vi "Barometer Bricklet Test.vi"() -> ()   [LabVIEW 2011]
uses:
  Classes/Device/Type Definitions/Callback Option.ctl
  Classes/IP Connection/IP Connection.lvclass
  Classes/Device/Device.lvclass
  Classes/Barometer Bricklet/Barometer Bricklet.lvclass
panel:
  out "appended array":bool[](array[boolean])
  out "x-y":u32
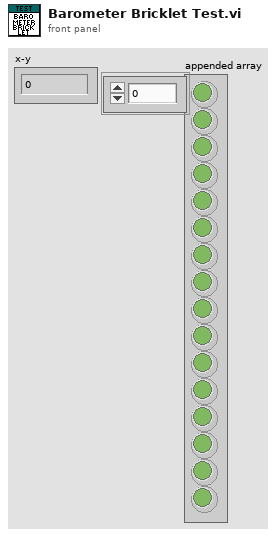
[diagram p1: front panel]
types:
  T1 = typedef "Tinkerforge.lvlib/Device.lvclass/Callback Option.ctl" = enum8{"CB off", "outside range", "inside range", "smaller", "greater"}
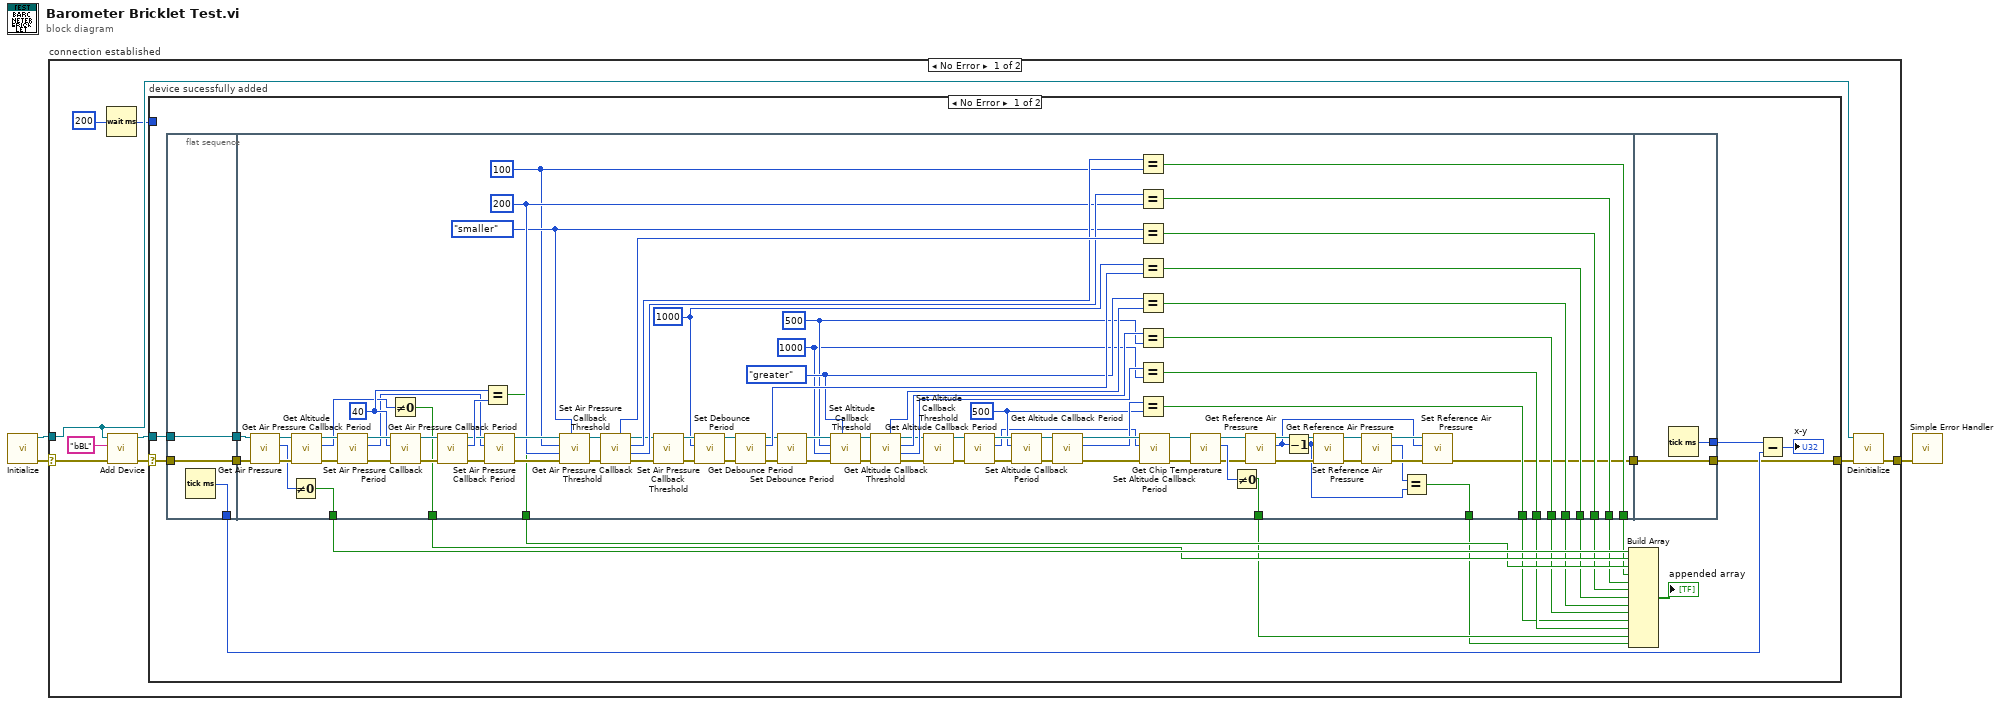
[diagram p0: block diagram]
diagram:
  n1 = call "Initialize.vi"() -> ("error out"=w1:errorcluster, "IP Connection out"=w3:refnum<class "IP Connection.lvclass">)  [unwired: 10 in]
  n2 = case "connection established" shown="No Error" w1 {
    selector: w1 -> [w8 w130]
    tunnel: w3 -> [w12 _]
    tunnel: [w4 w130] -> w2
    frame No Error {
      n3 = Wait (ms)(milliseconds to wait=u32 200) -> (millisecond timer value=w5:u32)
      n4 = call "Add Device.vi"("Error In"=w8, "Device UID"="bBL", "IP Connection"=w12) -> ("Error Out"=w7:errorcluster, "Barometer Bricklet"=w9:refnum<class "Barometer Bricklet.lvclass">)  [unwired: 7 in]
      n5 = case "device sucessfully added" shown="No Error" w7 {
        selector: w7 -> [w35 w129]
        tunnel: [w15 w129] -> w10
        tunnel: w9 -> [w34 _]
        tunnel: w5 -> [_ _]
        frame No Error {
          n6 = flat-sequence {
            tunnel: w34 -> [w37]
            tunnel: w35 -> [w38]
            tunnel: [w38] -> w32
            tunnel: [w37] -> w31
            tunnel: [w36] -> w29
            tunnel: [w43] -> w33
            tunnel: w32 -> [w126]
            tunnel: w31 -> [w125]
            tunnel: [w66] -> w27
            tunnel: [w65] -> w26
            tunnel: [w64] -> w25
            tunnel: [w63] -> w24
            tunnel: [w62] -> w23
            tunnel: [w61] -> w22
            tunnel: [w60] -> w21
            tunnel: [w59] -> w20
            tunnel: [w58] -> w19
            tunnel: [w57] -> w18
            tunnel: [w56] -> w17
            tunnel: [w42] -> w14
            tunnel: [w41] -> w13
            tunnel: [w128] -> w15
            tunnel: w33 -> [w128]
            tunnel: [w127] -> w30
            frame #0 {
              n7 = Tick Count (ms)() -> (millisecond timer value=w36:u32)
            }
            frame #1 {
              w68 = u32 500 ("period (0: off)")
              w80 = i16 1000 ("max")
              w82 = i16 500 ("min")
              w85 = Callback_Option."greater" ("Callback Option (off)")
              w95 = u32 1000 ("debounce (100)")
              w103 = i16 200 ("max")
              w88 = i16 100 ("min")
              w89 = Callback_Option."smaller" ("Callback Option (off)")
              w115 = u32 40
              n8 = call "Get Air Pressure.vi"("error in (no error)"=w126, "Barometer Bricklet in"=w125) -> ("error out"=w124:errorcluster, "Air Pressure"=w114:i32, "Barometer Bricklet out"=w123:refnum<class "Barometer Bricklet.lvclass">)  [unwired: 7 in]
              n9 = Not Equal To 0?(x=w114) -> (x != 0?=w66:bool)
              n10 = call "Get Altitude.vi"("error in (no error)"=w124, "Barometer Bricklet in"=w123) -> ("error out"=w122:errorcluster, "Altitude"=w113:i32, "Barometer Bricklet out"=w117:refnum<class "Barometer Bricklet.lvclass">)  [unwired: 7 in]
              n11 = call "Get Air Pressure Callback Period.vi"("error in (no error)"=w122, "Barometer Bricklet in"=w117) -> ("error out"=w121:errorcluster, "period"=w110:u32, "Barometer Bricklet out"=w118:refnum<class "Barometer Bricklet.lvclass">)  [unwired: 7 in]
              n12 = Not Equal To 0?(x=w113) -> (x != 0?=w65:bool)
              n13 = call "Set Air Pressure Callback Period.vi"("error in (no error)"=w121, "period (0: off)"=w115, "Barometer Bricklet in"=w118) -> ("error out"=w120:errorcluster, "Barometer Bricklet out"=w119:refnum<class "Barometer Bricklet.lvclass">)  [unwired: 7 in]
              n14 = call "Get Air Pressure Callback Period.vi"("error in (no error)"=w120, "Barometer Bricklet in"=w119) -> ("error out"=w112:errorcluster, "period"=w116:u32, "Barometer Bricklet out"=w111:refnum<class "Barometer Bricklet.lvclass">)  [unwired: 7 in]
              n15 = Equal?(x=w115, y=w116) -> (x = y?=w64:bool)
              n16 = call "Set Air Pressure Callback Period.vi"("error in (no error)"=w112, "period (0: off)"=w110, "Barometer Bricklet in"=w111) -> ("error out"=w109:errorcluster, "Barometer Bricklet out"=w107:refnum<class "Barometer Bricklet.lvclass">)  [unwired: 7 in]
              n17 = call "Set Air Pressure Callback Threshold.vi"("Callback Option (off)"=w89, "error in (no error)"=w109, "max"=w103, "min"=w88, "Barometer Bricklet in"=w107) -> ("error out"=w108:errorcluster, "Barometer Bricklet out"=w102:refnum<class "Barometer Bricklet.lvclass">)  [unwired: 5 in]
              n18 = call "Get Air Pressure Callback Threshold.vi"("error in (no error)"=w108, "Barometer Bricklet in"=w102) -> ("error out"=w101:errorcluster, "max"=w104:i32, "min"=w105:i32, "Barometer Bricklet out"=w100:refnum<class "Barometer Bricklet.lvclass">, "Callback Option"=w106:T1)  [unwired: 5 in]
              n19 = call "Set Air Pressure Callback Threshold.vi"("error in (no error)"=w101, "Barometer Bricklet in"=w100) -> ("error out"=w99:errorcluster, "Barometer Bricklet out"=w98:refnum<class "Barometer Bricklet.lvclass">)  [unwired: 8 in]
              n20 = call "Set Debounce Period.vi"("error in (no error)"=w99, "debounce (100)"=w95, "Barometer Bricklet in"=w98) -> ("error out"=w96:errorcluster, "Barometer Bricklet out"=w97:refnum<class "Barometer Bricklet.lvclass">)  [unwired: 7 in]
              n21 = call "Get Debounce Period.vi"("error in (no error)"=w96, "Barometer Bricklet in"=w97) -> ("error out"=w93:errorcluster, "debounce"=w94:u32, "Barometer Bricklet out"=w92:refnum<class "Barometer Bricklet.lvclass">)  [unwired: 7 in]
              n22 = call "Set Debounce Period.vi"("error in (no error)"=w93, "Barometer Bricklet in"=w92) -> ("error out"=w91:errorcluster, "Barometer Bricklet out"=w90:refnum<class "Barometer Bricklet.lvclass">)  [unwired: 8 in]
              n23 = call "Set Altitude Callback Threshold.vi"("Callback Option (off)"=w85, "error in (no error)"=w91, "max"=w80, "min"=w82, "Barometer Bricklet in"=w90) -> ("error out"=w87:errorcluster, "Barometer Bricklet out"=w86:refnum<class "Barometer Bricklet.lvclass">)  [unwired: 5 in]
              n24 = call "Get Altitude Callback Threshold.vi"("error in (no error)"=w87, "Barometer Bricklet in"=w86) -> ("error out"=w79:errorcluster, "max"=w81:i32, "min"=w83:i32, "Barometer Bricklet out"=w78:refnum<class "Barometer Bricklet.lvclass">, "Callback Option"=w84:T1)  [unwired: 5 in]
              n25 = call "Set Altitude Callback Threshold.vi"("error in (no error)"=w79, "Barometer Bricklet in"=w78) -> ("error out"=w77:errorcluster, "Barometer Bricklet out"=w76:refnum<class "Barometer Bricklet.lvclass">)  [unwired: 8 in]
              n26 = call "Get Altitude Callback Period.vi"("error in (no error)"=w77, "Barometer Bricklet in"=w76) -> ("error out"=w75:errorcluster, "period"=w67:u32, "Barometer Bricklet out"=w74:refnum<class "Barometer Bricklet.lvclass">)  [unwired: 7 in]
              n27 = call "Set Altitude Callback Period.vi"("error in (no error)"=w75, "period (0: off)"=w68, "Barometer Bricklet in"=w74) -> ("error out"=w72:errorcluster, "Barometer Bricklet out"=w71:refnum<class "Barometer Bricklet.lvclass">)  [unwired: 7 in]
              n28 = call "Get Altitude Callback Period.vi"("error in (no error)"=w72, "Barometer Bricklet in"=w71) -> ("error out"=w70:errorcluster, "period"=w69:u32, "Barometer Bricklet out"=w73:refnum<class "Barometer Bricklet.lvclass">)  [unwired: 7 in]
              n29 = Equal?(x=w105, y=w88) -> (x = y?=w63:bool)
              n30 = Equal?(x=w104, y=w103) -> (x = y?=w62:bool)
              n31 = Equal?(x=w89, y=w106) -> (x = y?=w61:bool)
              n32 = Equal?(x=w95, y=w94) -> (x = y?=w60:bool)
              n33 = Equal?(x=w85, y=w84) -> (x = y?=w59:bool)
              n34 = Equal?(x=w83, y=w82) -> (x = y?=w58:bool)
              n35 = Equal?(x=w81, y=w80) -> (x = y?=w57:bool)
              n36 = Equal?(x=w69, y=w68) -> (x = y?=w56:bool)
              n37 = call "Set Altitude Callback Period.vi"("error in (no error)"=w70, "period (0: off)"=w67, "Barometer Bricklet in"=w73) -> ("error out"=w55:errorcluster, "Barometer Bricklet out"=w54:refnum<class "Barometer Bricklet.lvclass">)  [unwired: 7 in]
              n38 = call "Get Chip Temperature.vi"("error in (no error)"=w55, "Barometer Bricklet in"=w54) -> ("error out"=w52:errorcluster, "temperature"=w53:i16, "Barometer Bricklet out"=w51:refnum<class "Barometer Bricklet.lvclass">)  [unwired: 7 in]
              n39 = Not Equal To 0?(x=w53) -> (x != 0?=w42:bool)
              n40 = call "Get Reference Air Pressure.vi"("error in (no error)"=w52, "Barometer Bricklet in"=w51) -> ("error out"=w50:errorcluster, "Reference Air Pressure"=w40:i32, "Barometer Bricklet out"=w49:refnum<class "Barometer Bricklet.lvclass">)  [unwired: 7 in]
              n41 = Decrement(x=w40) -> (x-1=w39:i32)
              n42 = call "Set Reference Air Pressure.vi"("error in (no error)"=w50, "Reference Air Pressure (0: acutal air pressure)"=w39, "Barometer Bricklet in"=w49) -> ("error out"=w47:errorcluster, "Barometer Bricklet out"=w46:refnum<class "Barometer Bricklet.lvclass">)  [unwired: 7 in]
              n43 = call "Get Reference Air Pressure.vi"("error in (no error)"=w47, "Barometer Bricklet in"=w46) -> ("error out"=w45:errorcluster, "Reference Air Pressure"=w44:i32, "Barometer Bricklet out"=w48:refnum<class "Barometer Bricklet.lvclass">)  [unwired: 7 in]
              n44 = Equal?(x=w44, y=w39) -> (x = y?=w41:bool)
              n45 = call "Set Reference Air Pressure.vi"("error in (no error)"=w45, "Reference Air Pressure (0: acutal air pressure)"=w40, "Barometer Bricklet in"=w48) -> ("error out"=w43:errorcluster)  [unwired: 7 in, 1 out]
            }
            frame #2 {
              n46 = Tick Count (ms)() -> (millisecond timer value=w127:u32)
            }
          }
          n47 = Build Array(w27, w26, w25, w24, w23, w22, w21, w20, w19, w17, w18, w14, w13) -> (→"appended array":bool[])
          n48 = Subtract(x=w30, y=w29) -> (x-y=→"x-y":u32)
        }
        frame Error {
        }
      }
      n49 = call "Deinitialize.vi"("error in (no error)"=w10, "IP Connection in"=w12) -> ("error out"=w4:errorcluster)  [unwired: 9 in]
    }
    frame Error {
    }
  }
  n50 = call <vilib>:"Simple Error Handler.vi"("error in (no error)"=w2) -> ()  [unwired: 4 in, 5 out]
